vi "Read One step per measurement.vi"(8 "error in (no error)":errorcluster, 11 "Stepper in":refnum<class "Stepper.lvclass">) -> (0 "error out":errorcluster, 2 "One step per measurement":bool, 3 "Stepper out":refnum<class "Stepper.lvclass">)   [LabVIEW 2021, in "Stepper.lvclass"]
uses:
  Stepper.lvclass
  Stepper.lvclass/Stepper.ctl
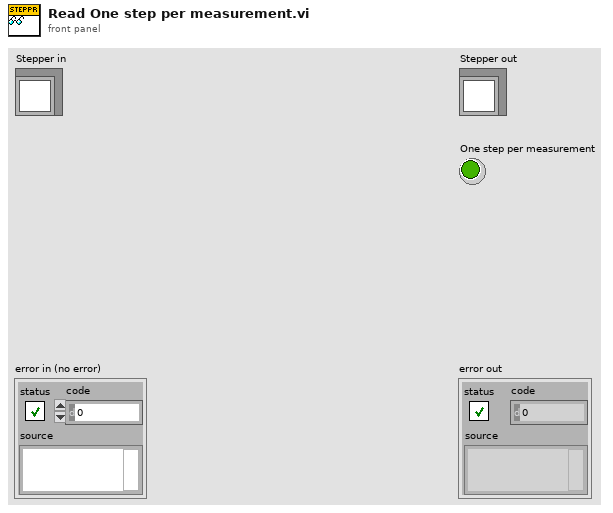
[diagram p1: front panel]
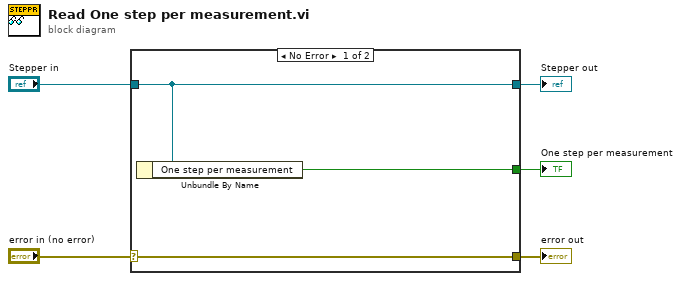
[diagram p0: block diagram]
diagram:
  n1 = case shown="No Error" "error in (no error)" {
    selector: "error in (no error)" -> [w8 w9]
    tunnel: [w8 w9] -> w4
    tunnel: [w7 w10] -> w2
    tunnel: "Stepper in" -> [w7 w10]
    tunnel: [w6 _] -> w1
    frame No Error {
      n2 = Unbundle By Name(w7) -> ("One step per measurement"=w6:bool)
    }
    frame Error {
    }
  }
  "error out" <- w4
  "Stepper out" <- w2
  "One step per measurement" <- w1
